vi "9068_6_9230.vi"() -> (2 "Device":T3={"Id"="5536b62219257936b04df4ed", "Name"="Bop9068", "DeviceType"="CMS-9068", "HardwareName"="", "IpAddress"="10.2.64.27", "HardwareInfo"=[{"Key"="Controller", "Value"="cRIO 9068"}, {"Key"="Slot 1", "Value"="NI 9230"}, {"Key"="Slot 2", "Value"="NI 9230"}, {"Key"="Slot 3", "Value"="NI 9230"}, {"Key"="Slot 4", "Value"="NI 9230"}, {"Key"="Slot 5", "Value"="NI 9230"}, {"Key"="Slot 6", "Value"="NI 9230"}, {"Key"="Slot 7", "Value"="NI 9205"}, {"Key"="Slot 8", "Value"=""}], "ApplicationType"="", "ApplicationVersion"="", "EquipmentIds"=[], "ConfigurationVersion"="2015-04-21T15:42:25.0576577-05:00", "ConfigurationBag"="", "Properties"=[{"Key"="FileMemoryTransferMode", "Value"="true"}, {"Key"="StreamMode", "Value"="InMemOrDisk"}, {"Key"="TdmsMemoryBlockSize", "Value"="8388608"}, {"Key"="TdmsMemoryStreamBlockSize", "Value"="1048576"}, {"Key"="ReconnectInterval", "Value"="30"}, {"Key"="PacketSizeKbytes", "Value"="16"}, {"Key"="InterPacketDelay", "Value"="0"}, {"Key"="FeatureSpeedCutoff", "Value"="120"}, {"Key"="SpeedReference", "Value"=""}, {"Key"="DataBlockLength", "Value"="4"}, {"Key"="DataBlockUnit", "Value"="Seconds"}, {"Key"="AcquisitionLength", "Value"="7"}, {"Key"="PreTriggerLength", "Value"="3"}, {"Key"="AcquisitionUnit", "Value"="Seconds"}, {"Key"="SampleRate", "Value"="4096"}], "DataGroups"=[{"Name"="Default", "ChannelIds"=["5536b62219257936b04df4ee", "5536b62219257936b04df4f3", "5536b62219257936b04df4f8", "5536b62219257936b04df4fd", "5536b62219257936b04df502", "5536b62219257936b04df507", "5536b62219257936b04df50c", "5536b62219257936b04df50d", "5536b62219257936b04df50e", "5536b62219257936b04df50f", "5536b62219257936b04df510", "5536b62219257936b04df511", "5536b62219257936b04df512", "5536b62219257936b04df513", "5536b62219257936b04df514", "5536b62219257936b04df515", "5536b62219257936b04df516", "5536b62219257936b04df517", "5536b62219257936b04df518", "5536b62219257936b04df519", "5536b62219257936b04df51a", "5536b62219257936b04df51b", "5536b62219257936b04df54c"], "GatingTrigger"={"Type"="", "Expression"="", "Conditions"=[]}, "OperatingStates"=[{"Id"="5536b62219257936b04df54a", "Name"="On", "StreamMode"=FALSE, "EnterTrigger"={"Type"="", "Expression"="", "Conditions"=[]}, "ExitTrigger"={"Type"="", "Expression"="", "Conditions"=[]}, "TagCollectionTrigger"={"Type"="", "Expression"="C1", "Conditions"=[{"Source"="5536b62219257936b04df54b", "Type"="TimespanSeconds", "Operator"="Greater", "CompareTo"="10", "DwellSeconds"=0.0}]}, "FileCollectionTrigger"={"Type"="", "Expression"="C1 OR C2", "Conditions"=[{"Source"="Cron", "Type"="Cron", "Operator"="Greater", "CompareTo"="0 0,1,2,3,4,5,6,7,8,9,10,11,12,13,14,15,16,17,18,19,20,21,22,23 * * * *", "DwellSeconds"=0.0}, {"Source"="5536b62219257936b04df521", "Type"="Double", "Operator"="Delta", "CompareTo"="1.0", "DwellSeconds"=0.0}]}, "Properties"=[{"Key"="AcquisitionLength", "Value"="7"}, {"Key"="PreTriggerLength", "Value"="3"}, {"Key"="AcquisitionUnit", "Value"="Seconds"}]}], "Properties"=[{"Key"="SpeedReference", "Value"="5536b62219257936b04df54c"}, {"Key"="DataBlockLength", "Value"="4"}, {"Key"="DataBlockUnit", "Value"="Seconds"}], "EquipmentIds"=[]}]}, 3 "system info":T1={"controller"={"vendorName"="National Instruments", "productName"="cRIO 9068", "serialNumber"="0191B106"}, "chassis"={"vendorName"="National Instruments", "productName"="NI cRIO-9068", "serialNumber"="0191B106"}, "modules"=[{"vendorName"="National Instruments", "productName"="NI 9230", "serialNumber"="01709BF5"}, {"vendorName"="National Instruments", "productName"="NI 9230", "serialNumber"="01840BD2"}, {"vendorName"="", "productName"="NI 9230", "serialNumber"=""}, {"vendorName"="", "productName"="NI 9230", "serialNumber"=""}, {"vendorName"="", "productName"="NI 9230", "serialNumber"=""}, {"vendorName"="", "productName"="NI 9230", "serialNumber"=""}, {"vendorName"="National Instruments", "productName"="NI 9205", "serialNumber"="0181B2F3"}, {"vendorName"="", "productName"="", "serialNumber"=""}]})   [LabVIEW 2017]
uses:
  <vilib>/addons/InsightCM/MessageBus/Base/controls/KeyValuePair.ctl
  <vilib>/addons/InsightCM/MessageBus/Base/KeyValuePairs.ctl
  <vilib>/addons/InsightCM/MessageBus/Base/controls/Condition.ctl
  <vilib>/addons/InsightCM/MessageBus/Base/controls/Trigger.ctl
  <vilib>/addons/InsightCM/MessageBus/Base/controls/OperatingState.ctl
  <vilib>/addons/InsightCM/MessageBus/Base/controls/DataGroup.ctl
  <vilib>/addons/InsightCM/MessageBus/Base/controls/Device.ctl
  <vilib>/addons/cRIODetectHW/control/cRIO Product Info.ctl
  <vilib>/addons/cRIODetectHW/cRIODetectHW.lvlib
  <vilib>/addons/cRIODetectHW/control/SystemHW.ctl
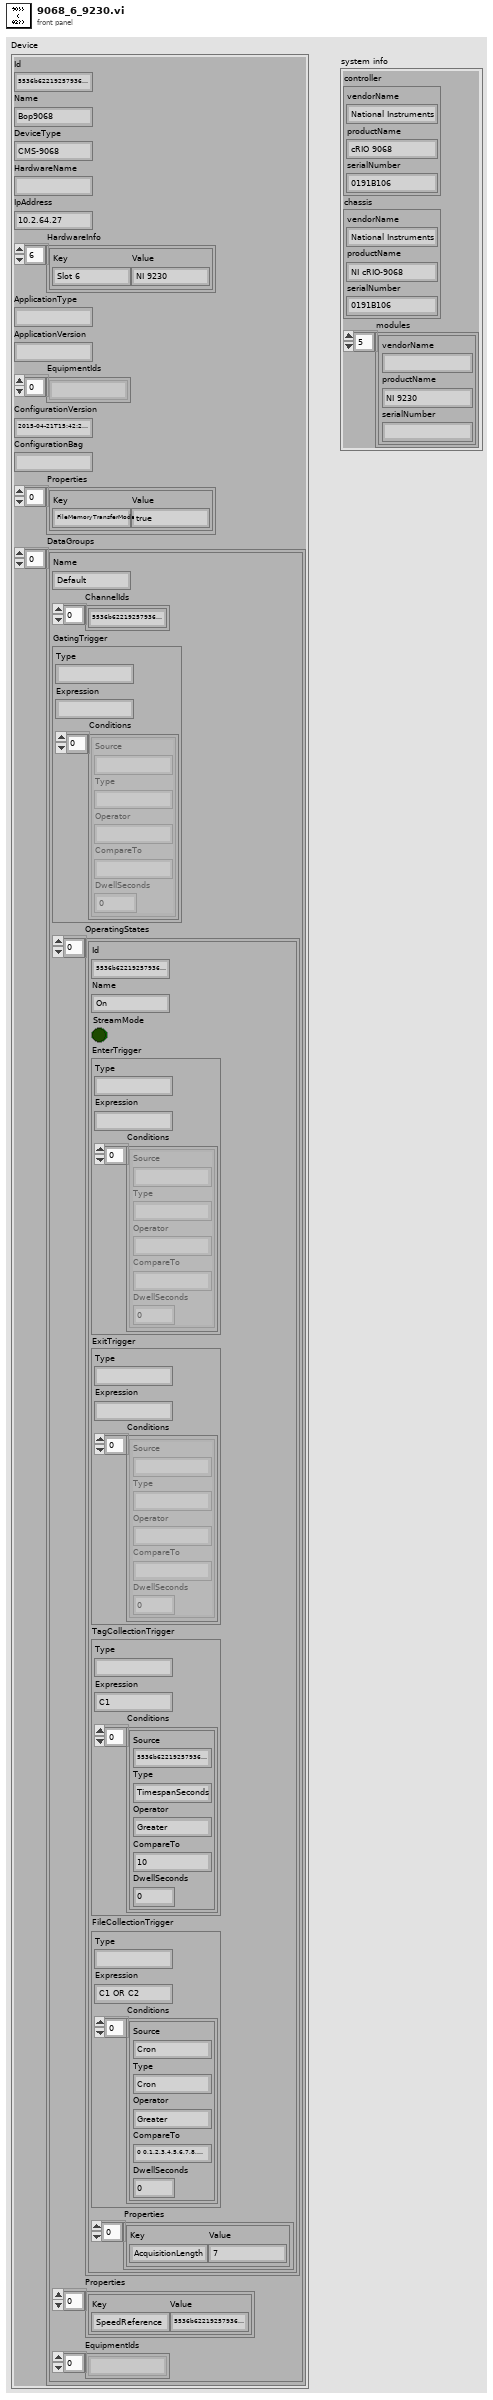
[diagram p1: front panel]
types:
  T1 = typedef "cRIODetectHW.lvlib/SystemHW.ctl" = cluster{"controller":T2, "chassis":T2, "modules":T2[]}
  T2 = typedef "cRIODetectHW.lvlib/cRIO Product Info.ctl" = cluster{"vendorName":string, "productName":string, "serialNumber":string}
  T3 = typedef "Device.ctl" = cluster{"Id":string, "Name":string, "DeviceType":string, "HardwareName":string, "IpAddress":string, "HardwareInfo":T4, "ApplicationType":string, "ApplicationVersion":string, "EquipmentIds":string[], "ConfigurationVersion":string, "ConfigurationBag":string, "Properties":T4, "DataGroups":T6[]}
  T4 = typedef "KeyValuePairs.ctl" = T5[]
  T5 = typedef "KeyValuePair.ctl" = cluster{"Key":string, "Value":string}
  T6 = typedef "DataGroup.ctl" = cluster{"Name":string, "ChannelIds":string[], "GatingTrigger":T7, "OperatingStates":T9[], "Properties":T4, "EquipmentIds":string[]}
  T7 = typedef "Trigger.ctl" = cluster{"Type":string, "Expression":string, "Conditions":T8[]}
  T8 = typedef "Condition.ctl" = cluster{"Source":string, "Type":string, "Operator":string, "CompareTo":string, "DwellSeconds":dbl}
  T9 = typedef "OperatingState.ctl" = cluster{"Id":string, "Name":string, "StreamMode":bool, "EnterTrigger":T7, "ExitTrigger":T7, "TagCollectionTrigger":T7, "FileCollectionTrigger":T7, "Properties":T4}
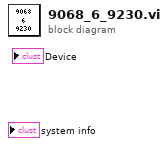
[diagram p0: block diagram]
diagram:
